vi "Write Eye and Eye Axis.vi"(8 "error in (no error)":errorcluster, 10 "Impulse Manager":refnum<class "Impulse Manager.lvclass">, 11 "Data Analyser Report in":refnum<class "Data Analyser Report.lvclass">) -> (0 "error out":errorcluster, 3 "Data Analyser Report out":refnum<class "Data Analyser Report.lvclass">)   [LabVIEW 2016, in "Data Analyser Report.lvclass"]
uses:
  Data Analyser Report.lvclass
  C:/Users/w.figtree/Desktop/Work/4. Projects/3. In Progress Engineering Projects/EMA/src/core/Classes/Excel Interface/Excel Sheet/Excel Sheet.lvclass
  Impulse Manager/Impulse Manager.lvclass
  Excel Interface/Excel Sheet/Write to Cell - String.vi
  Excel Interface/Excel Sheet/Excel Sheet.lvclass
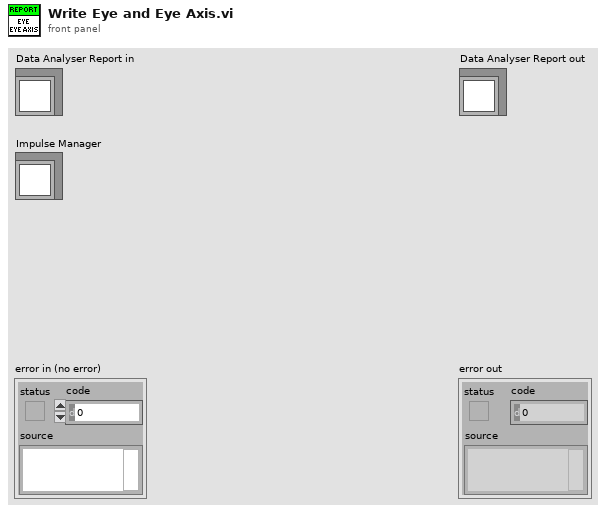
[diagram p1: front panel]
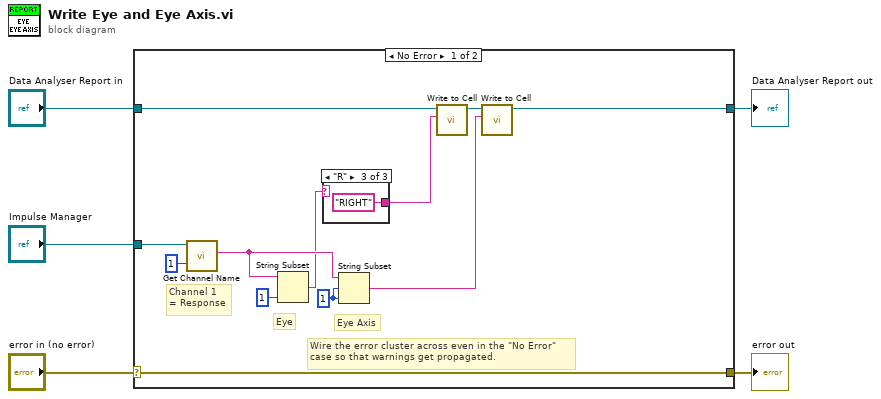
[diagram p0: block diagram]
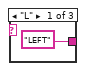
[diagram p2: hidden frame]
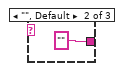
[diagram p3: hidden frame]
diagram:
  n1 = case shown="No Error" "error in (no error)" {
    selector: "error in (no error)" -> [w17 w22]
    tunnel: [w17 w22] -> w4
    tunnel: [w9 w21] -> w2
    tunnel: "Data Analyser Report in" -> [w11 w21]
    tunnel: "Impulse Manager" -> [w16 _]
    frame No Error {
      w12 = 1 ("length (rest)")
      # "Eye Axis"
      # "Channel 1 \n= Response"
      # "Eye"
      # "Wire the error cluster across even in the \"No Error\"\ncase so that warnings get propagated."
      n2 = call-dynamic "Get Channel Name.vi"("index"=1, "Impulse Manager in"=w16) -> ("Channel Name"=w13:string)  [unwired: 7 in, 2 out]
      n3 = String Subset(string=w13, length (rest)=1 ("length (rest)")) -> (substring=w8:string)  [unwired: 1 in]
      n4 = case shown="\"R\"" w8 {
        tunnel: ["LEFT" "" "RIGHT"] -> w7
        frame "L" {
        }
        frame "", Default {
        }
        frame "R" {
        }
      }
      n5 = String Subset(string=w13, offset (0)=w12, length (rest)=w12) -> (substring=w6:string)
      n6 = call-poly "Write to Cell.vi"("Value"=w7, "Excel Sheet in"=w11) -> ("Excel Sheet out"=w10:refnum<class "Data Analyser Report.lvclass">)  [unwired: 9 in]
      n7 = call-poly "Write to Cell.vi"("Value"=w6, "Excel Sheet in"=w10) -> ("Excel Sheet out"=w9:refnum<class "Data Analyser Report.lvclass">)  [unwired: 9 in]
    }
    frame Error {
    }
  }
  "error out" <- w4
  "Data Analyser Report out" <- w2
